vi "testCluster.vi"(8 "error in (no error)":errorcluster) -> (0 "error out":errorcluster)   [LabVIEW 2019, in "AssertionTest.lvlib" / "AssertEquals.lvlib"]
uses:
  AssertEquals.lvlib
  Assertion/Assertion.lvlib
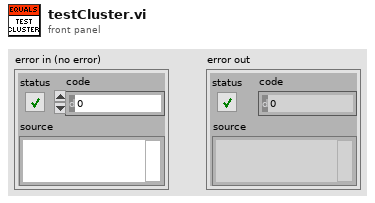
[diagram p1: front panel]
types:
  T1 = cluster{"String":string, "Numeric":i32, "Bool":bool}
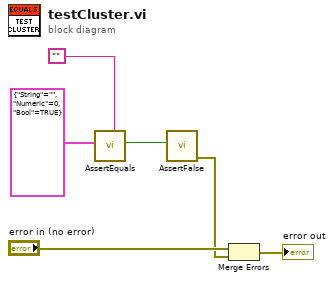
[diagram p0: block diagram]
diagram:
  n1 = call "AssertEquals.vi"("Expected"="", "Actual"=T1 {"String"="", "Numeric"=0, "Bool"=TRUE}) -> ("Result"=w4:bool)  [unwired: 8 in, 1 out]
  n2 = call "AssertFalse.vi"("Condition"=w4) -> ("error out"=w2:errorcluster)  [unwired: 9 in, 1 out]
  n3 = Merge Errors("error in (no error)", w2) -> (→"error out":errorcluster)
